vi "RGB-GS.vi"(8 "error in":errorcluster, 11 "Upload the Scan":path) -> (0 "error out":errorcluster, 2 "File Path":path, 3 "Refnum out":T1)   [LabVIEW 2024]
doc: "Image converstion from GRB to Gray scale"
uses:
  <vilib>/vision/Image Controls.llb/IMAQ Image.ctl
  <vilib>/vision/NI_Vision_Development_Module.lvlib
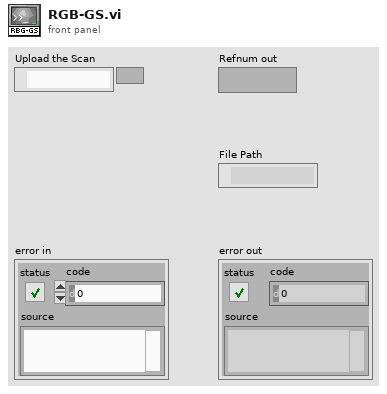
[diagram p1: front panel]
types:
  T1 = typedef "IMAQ Image.ctl" = refnum<image>
  T2 = typedef "Image Type" = u32
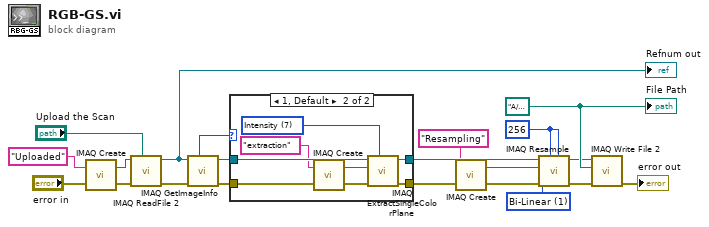
[diagram p0: block diagram]
diagram:
  w1 = u32 1 items=["Zero Order", "Bi-Linear", "Quadratic", "Cubic Spline"] ("Interpolation Type")
  w19 = path "A:/Siena/Bio-Tech Instrumentation/Stroke recovery time perdiction/temp image/1" ("File Path")
  w9 = 256 ("Y Resolution")
  n1 = call "IMAQ Create"("Image Name"="Uploaded", "error in (no error)"="error in") -> ("New Image"=w6:T1, "error out"=w5:errorcluster)  [unwired: 3 in]
  n2 = call "IMAQ ReadFile 2"("File Path"="Upload the Scan", "error in (no error)"=w5, "Image"=w6) -> ("error out"=w13:errorcluster, "Image Out"=w4:T1)  [unwired: 4 in, 3 out]
  "Refnum out" <- w4
  n3 = call "IMAQ GetImageInfo"("error in (no error)"=w13, "Image"=w4) -> ("error out"=w12:errorcluster, "Image Type"=w11:T2)  [unwired: 2 in, 6 out]
  n4 = case shown="1, Default" w11 {
    tunnel: w4 -> [w22 w30]
    tunnel: [w22 w28] -> w14
    tunnel: w12 -> [w21 w24]
    tunnel: [w21 w29] -> w15
    frame 0 {
    }
    frame 1, Default {
      w27 = 7 items=["Red", "Green", "Blue", "Hue", "Saturation", "Luminance", "Value", "Intensity"] ("Color Plane")
      n5 = call "IMAQ Create"("Image Name"="extraction", "error in (no error)"=w24) -> ("New Image"=w26:T1, "error out"=w23:errorcluster)  [unwired: 3 in]
      n6 = call "IMAQ ExtractSingleColorPlane"("Color Plane"=w27, "error in (no error)"=w23, "Image Dst"=w26, "Image Src"=w30) -> ("error out"=w29:errorcluster, "Image Dst Out"=w28:T1)  [unwired: 6 in]
    }
  }
  n7 = call "IMAQ Create"("Image Name"="Resampling", "error in (no error)"=w15) -> ("New Image"=w8:T1, "error out"=w10:errorcluster)  [unwired: 3 in]
  n8 = call "IMAQ Resample"("X Resolution"=w9, "Y Resolution"=w9, "error in (no error)"=w10, "Interpolation Type"=w1, "Image Dst"=w8, "Image Src"=w14) -> ("error out"=w16:errorcluster, "Image Dst Out"=w2:T1)  [unwired: 4 in]
  n9 = call-poly "IMAQ Write File 2"("error in (no error)"=w16, "File Path"=w19, "Image"=w2) -> ("error out"=→"error out":errorcluster)  [unwired: 7 in, 1 out]
  "File Path" <- w19
